vi "Get Running.vi"(8 "error in (no error)":errorcluster, 11 "2DArrayManager in":refnum<class "2DArrayManager.lvclass">) -> (0 "error out":errorcluster, 2 "Running":bool, 3 "2DArrayManager out":refnum<class "2DArrayManager.lvclass">)   [LabVIEW 2020, in "OOPanel.lvlib" / "2DArrayManager.lvclass"]
uses:
  2DArrayManager.lvclass
  2DArrayManager.lvclass/2DArrayManager.ctl
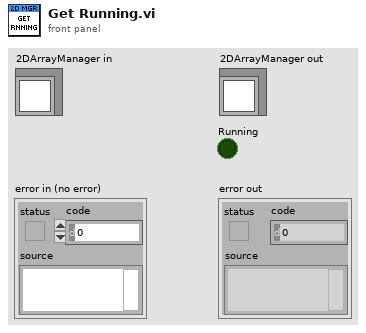
[diagram p1: front panel]
types:
  T1 = typedef "OOPanel.lvlib/2DArrayManager.lvclass/State Ref.ctl" = cluster{"Running":bool, "Borders":bool, "Total Height":dbl, "Background":u32, "V Scroll":bool, "H Scroll":bool}
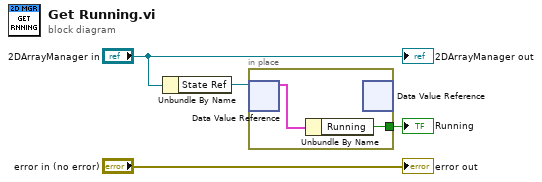
[diagram p0: block diagram]
diagram:
  n1 = Unbundle By Name("2DArrayManager in") -> ("State Ref"=w3:refnum<data-value>)
  n2 = in-place {
    in-place-border: [w5] -> w1
    n3 = in-place-dvr #1(w3) -> (w6:T1)  [unwired: 1 out]
    n4 = Unbundle By Name(w6) -> ("Running"=w5:bool)
    n5 = in-place-dvr #1() -> ()  [unwired: 1 in, 2 out]
  }
  "Running" <- w1
  "error out" <- "error in (no error)"
  "2DArrayManager out" <- "2DArrayManager in"
